vi "Create H File From Cpp.vi"(8 "error in":errorcluster, 11 "file in":path) -> (0 "error out":errorcluster, 3 "h file content":string)   [LabVIEW 2014]
doc: "This function traverse input .cpp file and is looking for functions prototypes. Then take them and put them into .h file."
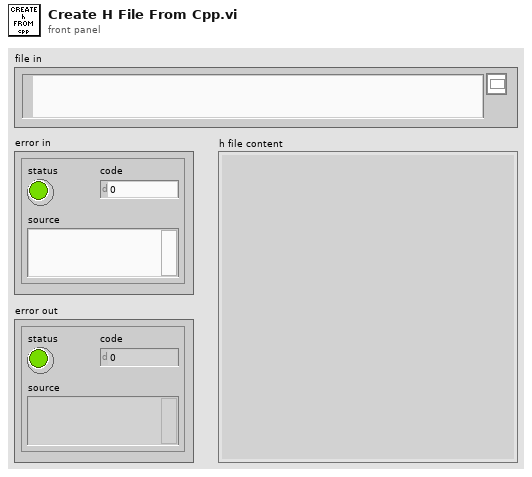
[diagram p1: front panel]
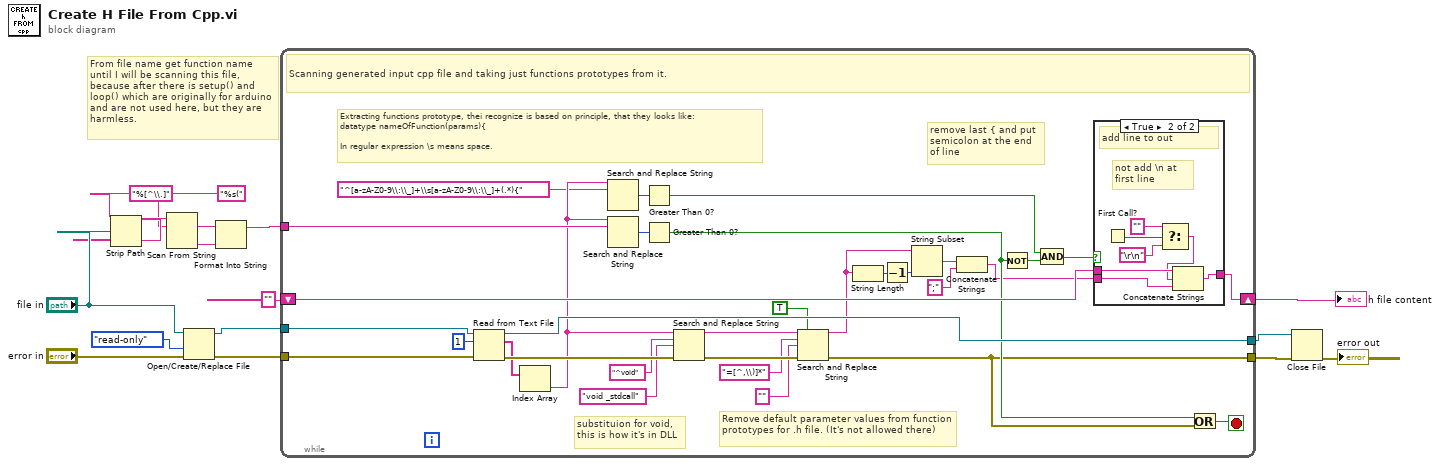
[diagram p0: block diagram]
diagram:
  # "From file name get function name until I will be scanning this file, because after there is setup() and loop() which are originally for arduino and are not used here, but they are harmless."
  n1 = Strip Path(path="file in") -> (name=w10:string)  [unwired: 1 out]
  n2 = Scan From String(format string="%[^\\.]", input string=w10) -> (output 1=w5:string)  [unwired: 3 in, 3 out]
  n3 = Open/Create/Replace File(file path (use dialog)="file in", error in="error in", access (0:read/write)=enum16{"read/write", "read-only", "write-only"}."read-only") -> (refnum out=w12:refnum<file>, error out=w13:errorcluster)  [unwired: 3 in, 1 out]
  n4 = Format Into String(format string="%s(", w5) -> (resulting string=w7:string)  [unwired: 2 in, 1 out]
  n5 = while {
    tunnel: w13 -> [w46]
    tunnel: w12 -> [w45]
    tunnel: [w20] -> w3
    tunnel: w7 -> [w34]
    shift-right: [w42] -> w4
    shift-left: "" -> [w41]
    tunnel: [w37] -> w1
    stop <- w43 stop-if-true
    # "Extracting functions prototype, thei recognize is based on principle, that they looks like:\ndatatype nameOfFunction(params){\n\nIn regular expression \\s means space."
    # "Remove default parameter values from function prototypes for .h file. (It's not allowed there)"
    # "remove last { and put semicolon at the end of line"
    # "substituion for void, this is how it's in DLL"
    # "Scanning generated input cpp file and taking just functions prototypes from it."
    n6 = Read from Text File(file (use dialog)=w45, count=1, error in=w46) -> (refnum out=w37:refnum<file>, text=w36:string[], error out=w40:errorcluster)  [unwired: 1 in, 1 out]
    n7 = Index Array(array=w36) -> (element=w33:string)  [unwired: 1 in]
    n8 = Search and Replace String(input string=w33, search string="^[a-zA-Z0-9\\:\\_]+\\s[a-zA-Z0-9\\:\\_]+(.*){") -> (number of replacements=w35:i32)  [unwired: 6 in, 3 out]
    n9 = Search and Replace String(input string=w33, search string=w34) -> (number of replacements=w44:i32)  [unwired: 6 in, 3 out]
    n10 = Greater Than 0?(x=w35) -> (x > 0?=w30:bool)
    n11 = Greater Than 0?(x=w44) -> (x > 0?=w29:bool)
    n12 = Search and Replace String(input string=w33, search string="^void", replace string="void _stdcall" ("search string"), error in=w40) -> (result string=w21:string, error out=w19:errorcluster)  [unwired: 4 in, 2 out]
    n13 = Search and Replace String(replace all?=TRUE ("replace all? (F)"), input string=w21, search string="=[^,\\)]*", replace string="" ("search string"), error in=w19) -> (result string=w22:string, error out=w20:errorcluster)  [unwired: 3 in, 2 out]
    n14 = String Length(string=w22) -> (length=w27:i32)
    n15 = Decrement(x=w27) -> (x-1=w26:i32)
    n16 = String Subset(string=w22, length (rest)=w26) -> (substring=w25:string)  [unwired: 1 in]
    n17 = Concatenate Strings(w25, ";" ("string")) -> (w24:string)
    n18 = Not(x=w29) -> (.not. x?=w28:bool)
    n19 = Compound Arithmetic op=AND(w30, w28) -> (w31:bool)
    n20 = case shown="True" w31 {
      tunnel: [w48 w55] -> w42
      tunnel: w41 -> [w48 w54]
      tunnel: w24 -> [_ w53]
      frame False {
      }
      frame True {
        # "not add \\n at first line"
        # "add line to out"
        n21 = First Call?() -> (First Call?: T/F=w51:bool)
        n22 = Select(t="", s=w51, f="\r\n") -> (s? t:f=w49:string)
        n23 = Concatenate Strings(w54, w49, w53) -> (w55:string)
      }
    }
    n24 = Or(x=w29, y=w20) -> (x .or. y?=w43:bool)
  }
  "h file content" <- w4
  n25 = Close File(refnum=w1, error in=w3) -> (error out=→"error out":errorcluster)  [unwired: 1 out]
